vi "Command Logging.vi"(8 "error in (no error)":errorcluster, 10 "TCP Network Connection in":refnum<k5>, 11 "String":string) -> (0 "error out":errorcluster)   [LabVIEW 2021]
doc: "Author: Scott Hannahs <sth@magnet.fsu.edu>\nCopyright 2018 Florida State University, All rights reserved."
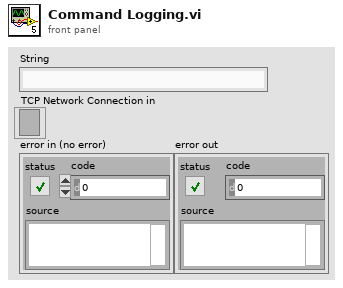
[diagram p1: front panel]
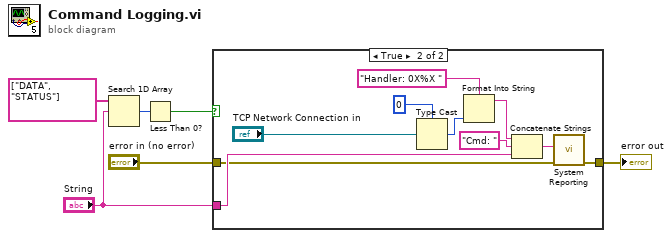
[diagram p0: block diagram]
diagram:
  n1 = Search 1D Array(1D array=string[] ["DATA", "STATUS"], element="String") -> (index of element=w4:i32)  [unwired: 1 in]
  n2 = Less Than 0?(x=w4) -> (x < 0?=w5:bool)
  n3 = case shown="True" w5 {
    tunnel: [w7 w15] -> w3
    tunnel: "String" -> [_ w14]
    tunnel: "error in (no error)" -> [w7 w13]
    frame False {
    }
    frame True {
      n4 = Type Cast(type=u32 0, x="TCP Network Connection in") -> (*(type *) &x=w8:u32)
      n5 = Format Into String(format string="Handler: 0X%X ", w8) -> (resulting string=w12:string)  [unwired: 2 in, 1 out]
      n6 = Concatenate Strings(w12, "Cmd: " ("string"), w14) -> (w17:string)
      n7 = call "System Reporting.vi"("Error In"=w13, "String"=w17) -> ("Error Out"=w15:errorcluster)  [unwired: 8 in, 1 out]
    }
  }
  "error out" <- w3
